vi "Canny Edge Detection Camera.vi"() -> ()   [LabVIEW 2018]
doc: "Canny Edge Detection Camera: This example is a Canny edge detection example of real-time sampling by camera, which is an image processing system using Canny edge detection algorithm. Canny edge detection is a classic edge detection algorithm designed to find strong edges in images and minimize false detections and false edges."
uses:
  vi.lib/VIRobotics/opencv_yiku/ctls/Size.ctl
  vi.lib/VIRobotics/opencv_yiku/Mat/Mat_8U/Mat_8U.lvclass
  D:/Program Files/company/National Instruments/LabVIEW 2018/vi.lib/addons/VIRobotics/opencv_yiku/Mat/Mat/Mat.lvclass
  vi.lib/VIRobotics/opencv_yiku/Cap/Cap.lvclass
  vi.lib/VIRobotics/opencv_yiku/opencv_yiku.lvlib
panel:
  out "channels":i32
  in  "sigmaX":dbl=5.0 format="%#_13g"
  in  "threshold2":dbl=10.0 format="%#_13g"
  in  "threshold1":dbl=30.0 format="%#_13g"
  in  "stop":bool
  out "pic":picture
  out "new pic":picture
  # "Overview: Demonstrates how to find edges with Canny Edge Detection\nRequirements: Windows.\nInstructions: \n1.Run the VI"
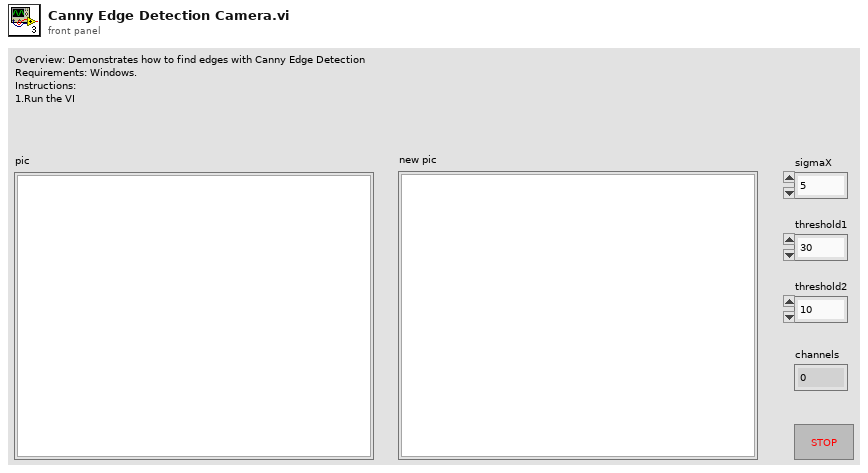
[diagram p1: front panel]
types:
  T1 = typedef "opencv_yiku.lvlib/Size.ctl" = cluster{"x":i32, "y":i32}
  T2 = enum16{"COLOR_BGR2BGRA", "COLOR_BGRA2BGR", "COLOR_BGR2RGBA", "COLOR_RGBA2BGR", "COLOR_BGR2RGB", "COLOR_BGRA2RGBA", "COLOR_BGR2GRAY", "COLOR_RGB2GRAY", "COLOR_GRAY2BGR", "COLOR_GRAY2BGRA"}
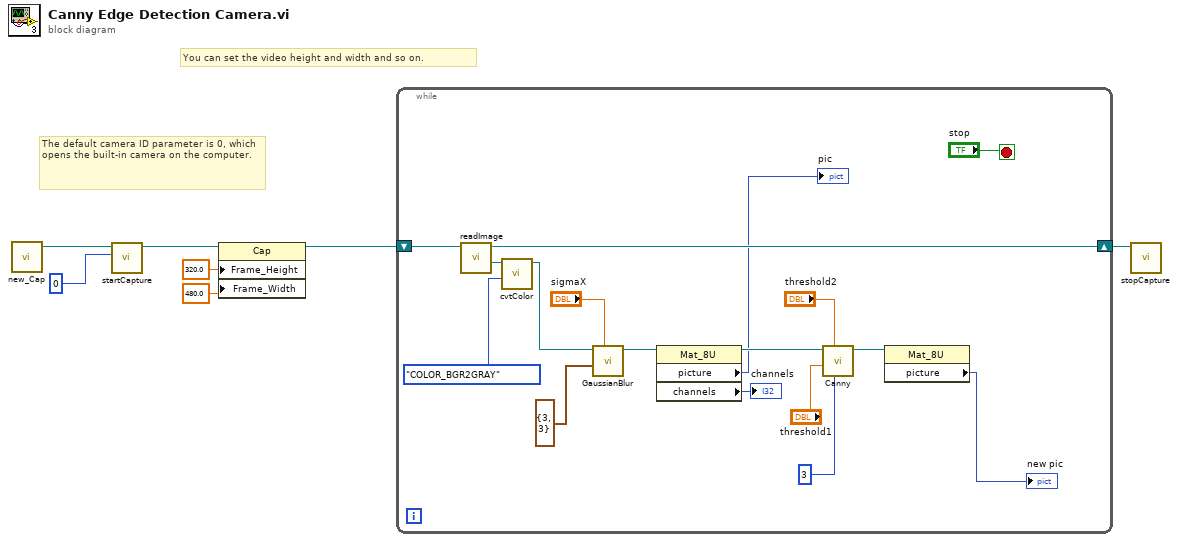
[diagram p0: block diagram]
diagram:
  # "You can set the video height and width and so on."
  # "The default camera ID parameter is 0, which opens the built-in camera on the computer."
  n1 = call "new_Cap.vi"() -> ("Cap out"=w7:refnum<class "Cap.lvclass">)  [unwired: 10 in, 1 out]
  n2 = call "startCapture.vi"("cameraID"=0, "Cap in"=w7) -> ("Cap out"=w4:refnum<class "Cap.lvclass">)  [unwired: 8 in, 1 out]
  n3 = property class="Cap"(reference=w4, "Frame_Height"=320.0, "Frame_Width"=480.0) -> (reference out=w3:refnum<class "Cap.lvclass">)  [unwired: 1 in, 1 out]
  n4 = while {
    shift-right: [w23] -> w5
    shift-left: w3 -> [w24]
    stop <- "stop" stop-if-true
    n5 = call "readImage.vi"("Cap in"=w24) -> ("Mat out"=w21:refnum<class "Mat_8U.lvclass">, "Cap out"=w23:refnum<class "Cap.lvclass">)  [unwired: 8 in, 1 out]
    n6 = call "cvtColor.vi"("dstCn"=T2."COLOR_BGR2GRAY", "src"=w21) -> ("src out"=w13:refnum<class "Mat_8U.lvclass">)  [unwired: 7 in, 2 out]
    n7 = call "GaussianBlur.vi"("sigmaX"="sigmaX", "Size"=T1 {"x"=3, "y"=3}, "Mat in"=w13) -> ("dst out"=w12:refnum<class "Mat_8U.lvclass">)  [unwired: 7 in, 1 out]
    n8 = property class="Mat_8U"(reference=w12) -> (reference out=w11:refnum<class "Mat_8U.lvclass">, "picture"=→"pic":picture, "channels"=→"channels":i32)  [unwired: 1 in, 1 out]
    n9 = call "Canny.vi"("apertureSize"=3, "threshold2"="threshold2", "threshold1"="threshold1", "Mat in"=w11) -> ("dst out"=w19:refnum<class "Mat_8U.lvclass">)  [unwired: 6 in, 1 out]
    n10 = property class="Mat_8U"(reference=w19) -> ("picture"=→"new pic":picture)  [unwired: 1 in, 2 out]
  }
  n11 = call "stopCapture.vi"("Cap in"=w5) -> ()  [unwired: 10 in, 1 out]
